vi "FGV2.vi"(5 "Enum":enum16{"Write", "Read"}(ring)=enum."Read", 8 "IN":T1) -> (1 "OUT":T1)   [LabVIEW 2016]
uses:
  Typedefs/FGV2_params.ctl
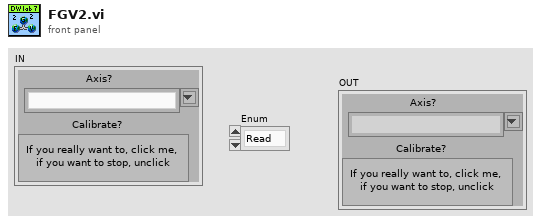
[diagram p1: front panel]
types:
  T1 = typedef "FGV2_params.ctl" = cluster{"Axis?":string, "Calibrate?":bool}
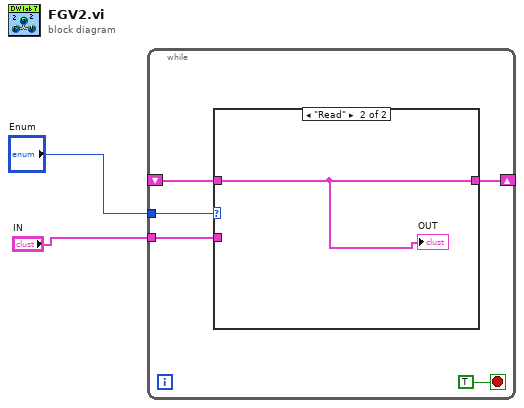
[diagram p0: block diagram]
diagram:
  n1 = while {
    tunnel: "IN" -> [w6]
    shift-right: [w5] -> _
    shift-left: _ -> [w4]
    tunnel: "Enum" -> [w3]
    stop <- TRUE stop-if-true
    n2 = case shown="\"Read\"" w3 {
      tunnel: w6 -> [w8 _]
      tunnel: [w8 w9] -> w5
      tunnel: w4 -> [_ w9]
      frame "Write", Default {
      }
      frame "Read" {
        "OUT" <- w9
      }
    }
  }
